vi "exec.vi"(8 "error in (no error)":errorcluster, 10 "context":refnum<class "Context.lvclass">, 11 "StartAutomatedTest in":refnum<class "StartAutomatedTest.lvclass">) -> (0 "error out":errorcluster, 2 "context 2":refnum<class "Context.lvclass">, 3 "StartAutomatedTest out":refnum<class "StartAutomatedTest.lvclass">)   [LabVIEW 2013, in "StartAutomatedTest.lvclass"]
uses:
  StartAutomatedTest.lvclass
  Context/Context.lvclass
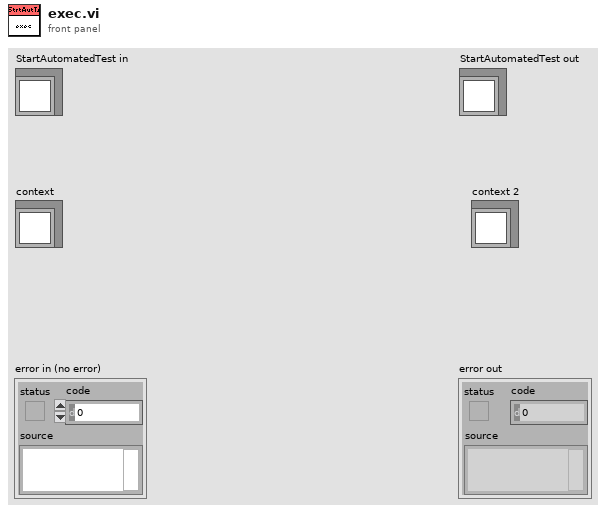
[diagram p1: front panel]
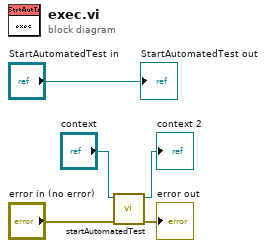
[diagram p0: block diagram]
diagram:
  n1 = call "startAutomatedTest.vi"("error in (no error)"="error in (no error)", "Context in"="context") -> ("error out"=→"error out":errorcluster, "Context out"=→"context 2":refnum<class "Context.lvclass">)  [unwired: 8 in]
  "StartAutomatedTest out" <- "StartAutomatedTest in"
